vi "getAbsolutePosition.vi"(8 "error in":errorcluster, 10 "axis":i32, 11 "connection ID":refnum<k5>) -> (0 "error out":errorcluster, 1 "position":dbl, 2 "axis_out":i32, 3 "connection ID":refnum<k5>)   [LabVIEW 2016]
doc: "The absolute position information is estimated at the measurement initialization procedure."
panel:
  out "params_cluster":cluster{"axis":i32}
  in  "Params_cluster":cluster{"integer":i32}
  in  "results_cluster":cluster{"warningNo":i32, "position":dbl}
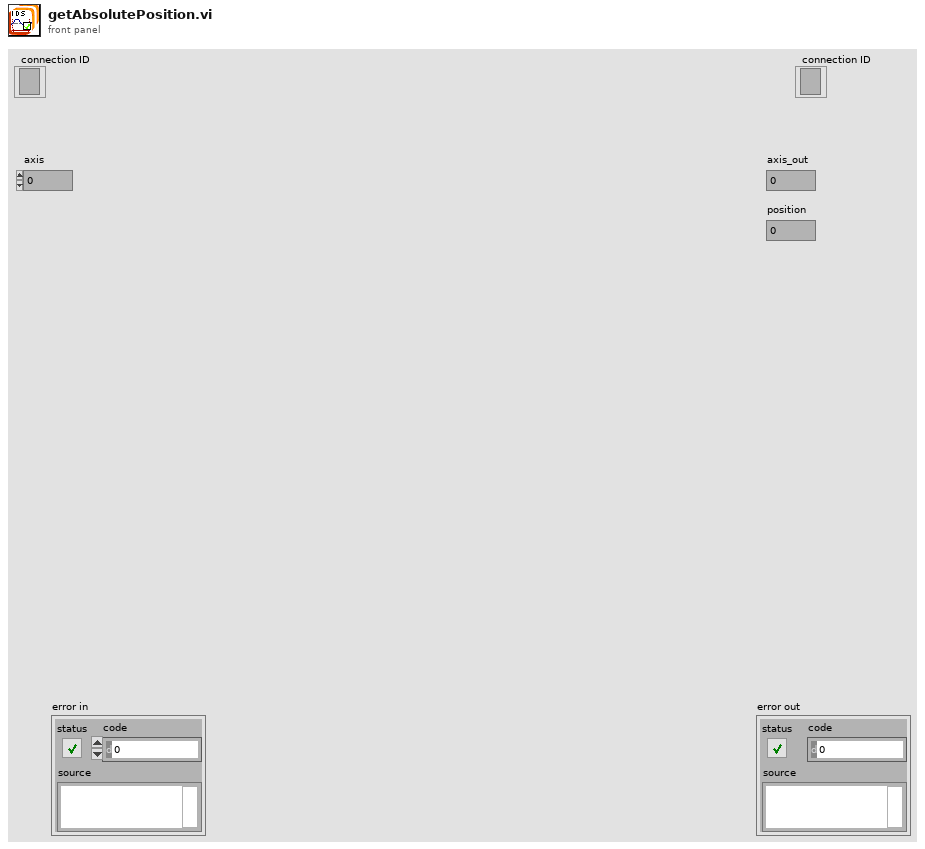
[diagram p1: front panel]
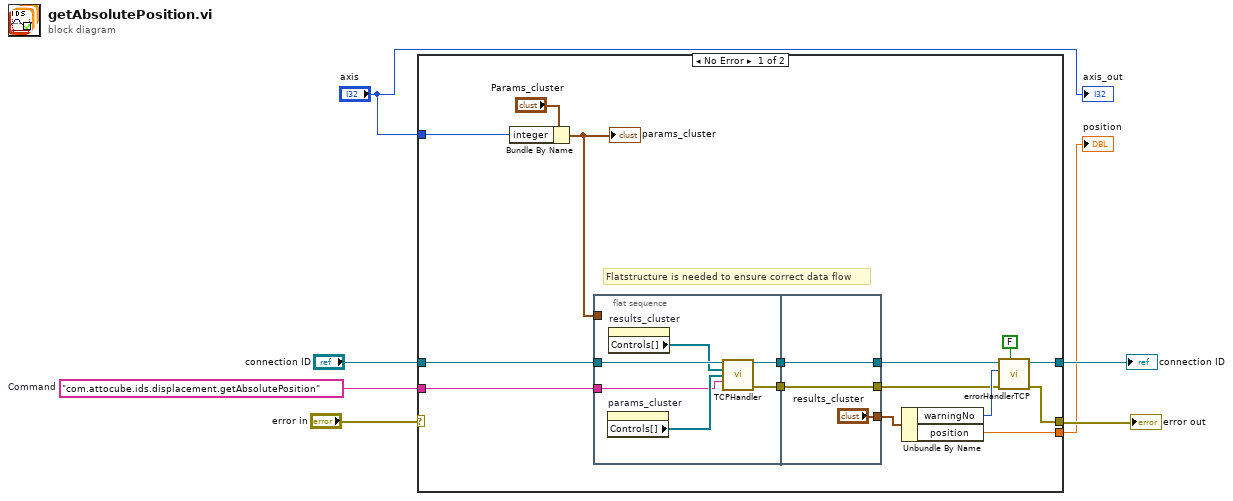
[diagram p0: block diagram]
diagram:
  w3 = "com.attocube.ids.displacement.getAbsolutePosition"  # Command
  n1 = case shown="No Error" "error in" {
    selector: "error in" -> [_ w33]
    tunnel: [w20 w33] -> w7
    tunnel: [w22 w32] -> w6
    tunnel: "connection ID" -> [w19 w32]
    tunnel: w3 -> [w13 _]
    tunnel: "axis" -> [w9 _]
    tunnel: [w8 _] -> w1
    frame No Error {
      # "Flatstructure is needed to ensure correct data flow"
      n2 = Bundle By Name(cluster="Params_cluster", "integer"=w9) -> (w10:cluster{"integer":i32})
      "params_cluster" <- w10
      n3 = flat-sequence {
        tunnel: [w27] -> w15
        tunnel: w19 -> [w28]
        tunnel: w13 -> [w24]
        tunnel: [w23] -> w11
        tunnel: w10 -> [_]
        tunnel: ["results_cluster"] -> w16
        tunnel: [w31] -> w18
        tunnel: w15 -> [w31]
        tunnel: [w29] -> w12
        tunnel: w11 -> [w29]
        frame #0 {
          n4 = property on="params_cluster" class="Clust (strict)"() -> ("Controls[]"=w25:refnum<vi>[])  [unwired: 2 in, 2 out]
          n5 = property on="results_cluster" class="Clust (strict)"() -> ("Controls[]"=w26:refnum<vi>[])  [unwired: 2 in, 2 out]
          n6 = call "TCPHandler.vi"("connection ID"=w28, "results_cluster"=w26, "params_cluster"=w25, "method"=w24) -> ("connection ID"=w27:refnum<k5>, "error"=w23:errorcluster)  [unwired: 8 in, 2 out]
        }
        frame #1 {
        }
      }
      n7 = Unbundle By Name(w16) -> ("warningNo"=w17:i32, "position"=w8:dbl)
      n8 = call "errorHandlerTCP.vi"("show popup"=FALSE, "error in"=w12, "error number"=w17, "connection ID"=w18) -> ("error out"=w20:errorcluster, "connection ID"=w22:refnum<k5>)  [unwired: 6 in]
    }
    frame Error {
    }
  }
  "error out" <- w7
  "connection ID" <- w6
  "position" <- w1
  "axis_out" <- "axis"
